vi "Kinect Video Controller.vi"() -> (1 "y":dbl, 2 "Distance":dbl, 3 "x":dbl)   [LabVIEW 2015]
uses:
  subVIs/Video Resolution Control.ctl
  subVIs/Video Format Control.ctl
  subVIs/Depth Format Control.ctl
  subVIs/Depth Resolution Control.ctl
  subVIs/Led Control.ctl
  subVIs/Log Level Control.ctl
panel:
  out "error out":errorcluster
  in  "Led Option":T1
  in  "Video and Depth config":T6={"Video Resolution"=enum."FREENECT_RESOLUTION_MEDIUM", "Video Format"=enum."FREENECT_VIDEO_RGB", "Depth Format"=enum."FREENECT_DEPTH_11BIT", "Depth Resolution"=enum."FREENECT_RESOLUTION_MEDIUM"}
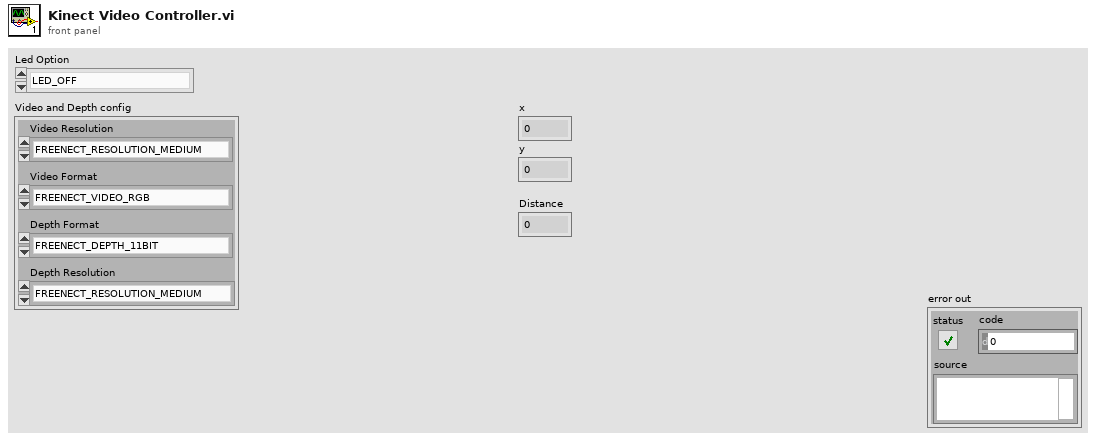
[diagram p1: front panel]
types:
  T1 = typedef "Led Control.ctl" = enum32{"LED_OFF", "LED_GREEN", "LED_RED", "LED_YELLOW", "LED_BLINK_GREEN", "LED_BLINK_GREEN2", "LED_BLINK_RED_YELLOW"}
  T2 = typedef "Video Resolution Control.ctl" = enum32{"FREENECT_RESOLUTION_LOW", "FREENECT_RESOLUTION_MEDIUM", "FREENECT_RESOLUTION_HIGH"}
  T3 = typedef "Video Format Control.ctl" = enum32{"FREENECT_VIDEO_RGB", "FREENECT_VIDEO_BAYER", "FREENECT_VIDEO_IR_8BIT", "FREENECT_VIDEO_IR_10BIT", "FREENECT_VIDEO_IR_10BIT_PACKED", "FREENECT_VIDEO_YUV_RGB", "FREENECT_VIDEO_YUV_RAW"}
  T4 = typedef "Depth Format Control.ctl" = enum32{"FREENECT_DEPTH_11BIT", "FREENECT_DEPTH_10BIT", "FREENECT_DEPTH_11BIT_PACKED", "FREENECT_DEPTH_10BIT_PACKED", "FREENECT_DEPTH_REGISTERED", "FREENECT_DEPTH_MM"}
  T5 = typedef "Depth Resolution Control.ctl" = enum16{"FREENECT_RESOLUTION_TINY", "FREENECT_RESOLUTION_LOW", "FREENECT_RESOLUTION_MEDIUM"}
  T6 = cluster{"Video Resolution":T2, "Video Format":T3, "Depth Format":T4, "Depth Resolution":T5}
  T7 = typedef "Log Level Control.ctl" = enum32{"FREENECT_LOG_FATAL", "FREENECT_LOG_ERROR", "FREENECT_LOG_WARNING", "FREENECT_LOG_NOTICE", "FREENECT_LOG_INFO", "FREENECT_LOG_DEBUG", "FREENECT_LOG_SPEW", "FREENECT_LOG_FLOOD"}
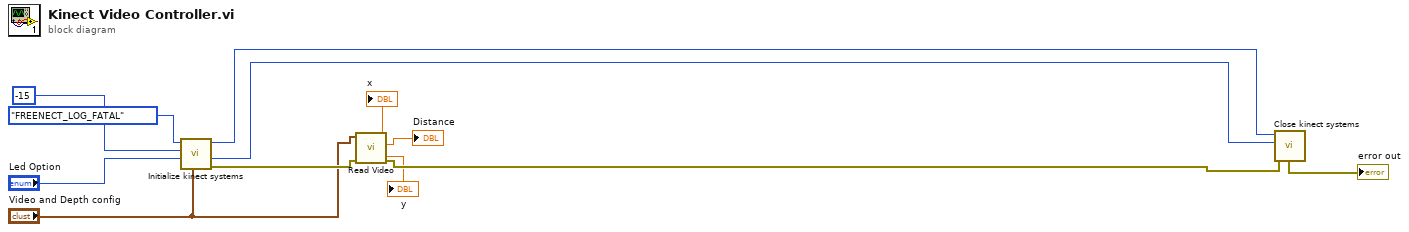
[diagram p0: block diagram]
diagram:
  n1 = call "Initialize kinect systems.vi"("Video and Depth config"="Video and Depth config", "Led Option"="Led Option", "tilt degree"=-15, "Log Level"=Log_Level_Control."FREENECT_LOG_FATAL") -> ("error out"=w6:errorcluster, "Kinect Handle"=w8:i64, "Video Handle out"=w9:i64)  [unwired: 4 in, 1 out]
  n2 = call "Read Video.vi"("error in (no error)"=w6, "input cluster"="Video and Depth config") -> ("error out"=w5:errorcluster, "Distance O"=→"Distance":dbl, "y"=→"y":dbl, "x"=→"x":dbl)  [unwired: 2 in, 2 out]
  n3 = call "Close kinect systems.vi"("error in (no error)"=w5, "Kinect Handle"=w8, "Video handle in"=w9) -> ("error out"=→"error out":errorcluster)  [unwired: 8 in]
